vi "Command_Goto.vi"(2 "node":string, 3 "Side":T1, 4 "Desired Position":sgl=100.0 min=0 max=100, 6 "error in":errorcluster) -> (5 "error out":errorcluster)   [LabVIEW 2010]
doc: "This will open or close the gripper to a specific position"
uses:
  <userlib>/ROSforLV_0.1/ROS/Code/SubVIs/BaxterSide.ctl
  <userlib>/ROSforLV_0.1/ROS/MessageBuilding/Primitives/subs/float32Scalar.vi
panel:
  # "Gripper position is from [0.0-100.0] [close-open]"
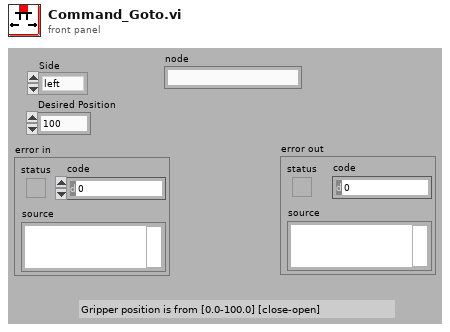
[diagram p1: front panel]
types:
  T1 = typedef "BaxterSide.ctl" = enum16{"left", "right"}
  T2 = typedef "_ROSControl.ctl" = cluster{"topic port":u16, "Node":string, "topic":string, "type":string, "node port":u32, "error ":errorcluster, "Direction":T3, "APIs":string[]}
  T3 = typedef "_ROSDirection.ctl" = enum16{"Node", "Publisher", "Subscriber", "Service Client"}
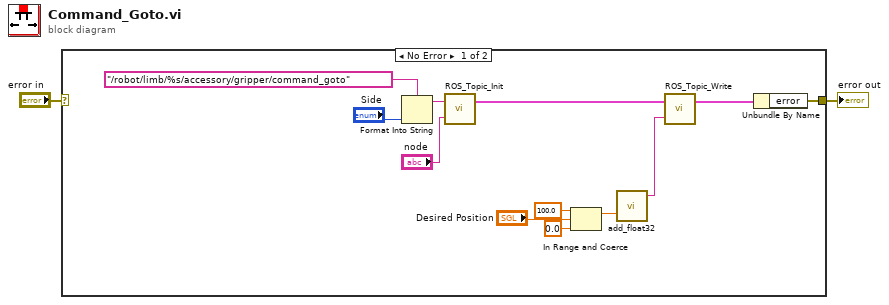
[diagram p0: block diagram]
diagram:
  n1 = case shown="No Error" "error in" {
    selector: "error in" -> [_ w15]
    tunnel: [w12 w15] -> w2
    frame No Error {
      n2 = Format Into String(format string="/robot/limb/%s/accessory/gripper/command_goto" ("topic"), "Side") -> (resulting string=w9:string)  [unwired: 2 in, 1 out]
      n3 = call <userlib>:"ROS_Topic_Init.vi"("node"="node", "topic"=w9) -> ("ROS out"=w14:T2)  [unwired: 1 in]
      n4 = In Range and Coerce(upper limit=sgl 100.0, x="Desired Position", lower limit=sgl 0.0) -> (coerced(x)=w3:sgl)  [unwired: 1 out]
      n5 = call-poly <userlib>:"add_float32.vi"("Numeric"=w3) -> ("msg out"=w8:string)  [unwired: 4 in]
      n6 = call <userlib>:"ROS_Topic_Write.vi"("Msg in"=w8, "ROS in"=w14) -> ("ROS out"=w13:T2)  [unwired: 1 in]
      n7 = Unbundle By Name(w13) -> ("error"=w12:errorcluster)
    }
    frame Error {
    }
  }
  "error out" <- w2
